vi "VAI Init ADC.vi"(7 "Period":u16, 8 "error in (no error)":errorcluster, 9 "Channel":u8, 10 "DevIndex":i32, 11 "DevType":i32) -> (0 "error out":errorcluster, 3 "function return":i32)   [LabVIEW 2012, in "ControlADC.lvlib"]
doc: "int WINAPI VAI_InitADC(int DevType, int DevIndex, unsigned char Channel, unsigned short Period);"
uses:
  ControlADC.lvlib
  Ginkgo_Driver.dll
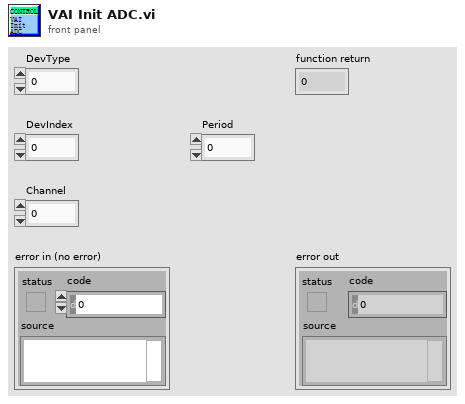
[diagram p1: front panel]
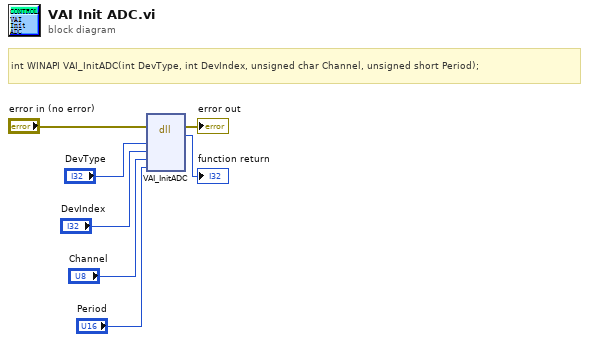
[diagram p0: block diagram]
diagram:
  # "int WINAPI VAI_InitADC(int DevType, int DevIndex, unsigned char Channel, unsigned short Period);"
  n1 = dll-call lib="E:/Project/vt_ginkgo/truck/Ginkgo Driver/vs2010/Ginkgo_USB-I2C_API_v2.0.3.0/lib/labview_32bit/ControlADC/Ginkgo_Driver.*" fn="VAI_InitADC"(error in="error in (no error)", "DevType"="DevType", "DevIndex"="DevIndex", "Channel"="Channel", "Period"="Period") -> (error out=→"error out":errorcluster, →"function return":i32)  [unwired: 6 in, 1 out]
